vi "XNET Read (State Time Current).vi"(0 "session in":refnum<k21>, 11 "error in (no error)":errorcluster) -> (4 "session out":refnum<k21>, 6 "local time current":timestamp, 13 "network synced":bool, 14 "network time current":timestamp, 15 "error out":errorcluster)   [LabVIEW 2018]
doc: "Reads the current interface timestamp using an XNET session. The time is returned as a LabVIEW absolute timestamp. <B>local time communicating</B> uses the local timescale. <B>network time communicating</B> and <B>network synced</B> are applicable only for an Ethernet interface."
uses:
  nixlvapi.dll
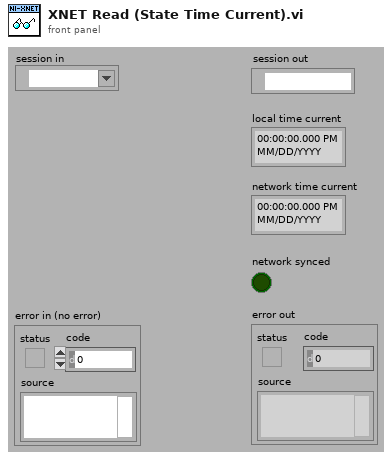
[diagram p1: front panel]
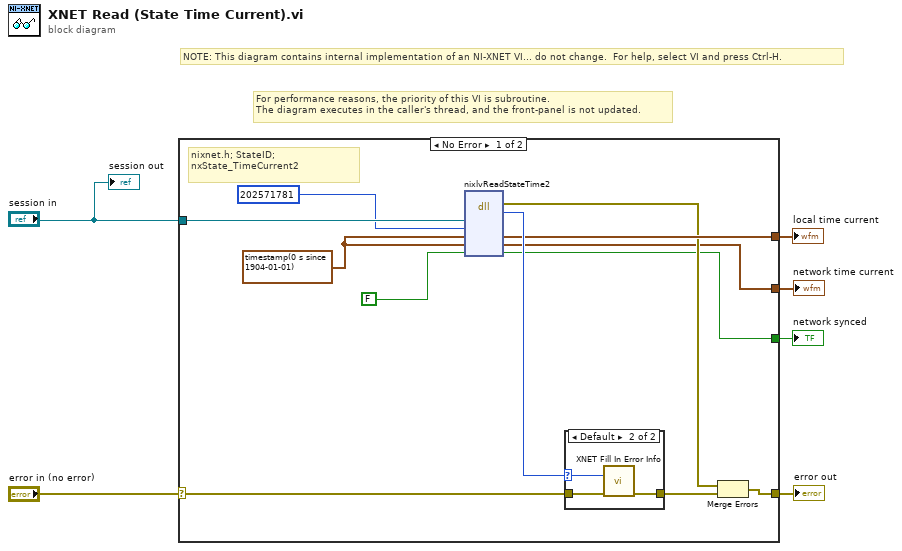
[diagram p0: block diagram]
diagram:
  # "For performance reasons, the priority of this VI is subroutine.\nThe diagram executes in the caller's thread, and the front-panel is not updated."
  # "NOTE: This diagram contains internal implementation of an NI-XNET VI... do not change.  For help, select VI and press Ctrl-H."
  n1 = case shown="No Error" "error in (no error)" {
    selector: "error in (no error)" -> [w17 w23]
    tunnel: "session in" -> [w18 _]
    tunnel: [w12 w23] -> w6
    tunnel: [w14 _] -> w3
    tunnel: [w9 _] -> w2
    tunnel: [w7 _] -> w1
    frame No Error {
      w10 = timestamp(0 s since 1904-01-01) ("time communication")
      # "nixnet.h; StateID;\nnxState_TimeCurrent2"
      n2 = dll-call lib="nixlvapi.*" fn="nixlvReadStateTime2"("sessionRef"=w18, "stateID"=u32 202571781 ("ParamOut"), "localTime"=w10, "networkTime"=w10, "networkSynced"=FALSE ("network synced")) -> (error out=w11:errorcluster, "return type"=w15:i32, "localTime"=w14:timestamp, "networkTime"=w9:timestamp, "networkSynced"=w7:bool)  [unwired: 4 in, 2 out]
      n3 = case shown="Default" w15 {
        selector: w15 -> [_ w20]
        tunnel: w17 -> [w19 w21]
        tunnel: [w19 w22] -> w16
        frame 0 {
        }
        frame Default {
          n4 = call "XNET Fill In Error Info.vi"("status code"=w20, "error in"=w21) -> ("error out"=w22:errorcluster)  [unwired: 13 out]
        }
      }
      n5 = Merge Errors(w11, w16) -> (w12:errorcluster)
    }
    frame Error {
    }
  }
  "error out" <- w6
  "local time current" <- w3
  "network time current" <- w2
  "network synced" <- w1
  "session out" <- "session in"
